vi "loop counter.vi"() -> (7 "Count":i32)   [LabVIEW 2017]
doc: "Counts the number of iterations inside a case structure of a loop."
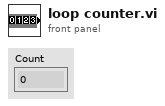
[diagram p1: front panel]
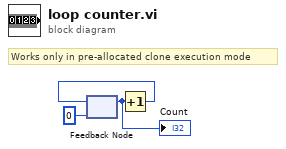
[diagram p0: block diagram]
diagram:
  # "Works only in pre-allocated clone execution mode"
  n1 = feedback #1(0) -> (w2:i32)
  "Count" <- w2
  n2 = Increment(x=w2) -> (x+1=w3:i32)
  n3 = feedback-in #1(w3) -> ()
